vi "Create Test Configuration.vi"(9 "Channel Classification":T1[](array[typedef])=[enum."input data", enum."output data", enum."input data", enum."output data"], 10 "Modbus Type":T2[](array[typedef])=[enum."Holding Registers", enum."Holding Registers", enum."Coils", enum."Coils"], 11 "Data Type":T3[](array[typedef])=[enum."U16", enum."U16", enum."Boolean", enum."Boolean"]) -> (0 "error out":errorcluster, 1 "Names":string[](array[string]), 2 "Channels":refnum<class "Modbus Module Channel.lvclass">[](array[class]), 3 "Module configuration":refnum<class "Modbus Module configuration.lvclass">)   [LabVIEW 2015, in "Modbus Tests.lvlib"]
uses:
  Modbus Tests.lvlib
  module/configuration/Modbus Module configuration.lvclass
  module/module channel/Modbus Module Channel.lvclass
  <vilib>/NI/Tag Bus/tag/Data Type.ctl
  module/module channel/data bank type.ctl
  <vilib>/NI/Tag Bus Module Framework/channel/channel classification.ctl
  <vilib>/NI/Tag Bus/tag/tag descriptor.lvclass/tag descriptor.ctl
  module/module channel/Modbus Module Channel.lvclass/Modbus Module Channel.ctl
  <vilib>/NI/Tag Bus Module Framework/channel/TBM channel.lvclass/TBM channel.ctl
  <vilib>/NI/Tag Bus/tag/write data type.vi
  module/module channel/Write modbus type.vi
  module/module channel/Write starting address.vi
  <vilib>/NI/Tag Bus Module Framework/channel/Write channel classification.vi
  <vilib>/NI/Tag Bus/tag/write tag name.vi
  <vilib>/NI/Configuration Framework/serializable configuration/NISE_CEF_serializable configuration.lvclass
  <vilib>/NI/Tag Bus/tag/tag descriptor.lvclass
  <vilib>/NI/Tag Bus Module Framework/channel/TBM channel.lvclass
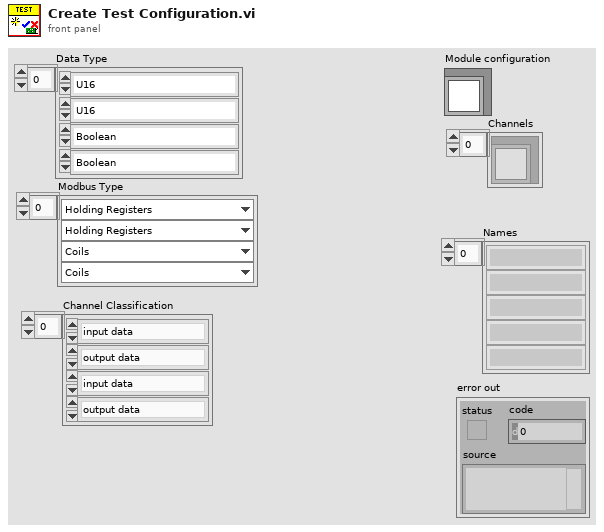
[diagram p1: front panel]
types:
  T1 = typedef "TBM channel.lvclass/channel classification.ctl" = enum16{"input data", "output data", "processing parameter", "processing result"}
  T2 = typedef "Modbus Module Channel.lvclass/data bank type.ctl" = enum16{"Coils", "Discrete Inputs", "Input Registers", "Holding Registers"}
  T3 = typedef "tag bus.lvlib/tag descriptor.lvclass/Data Type.ctl" = enum16{"Double", "Single", "I64", "I32", "I16", "I8", "U64", "U32", "U16", "U8", "Boolean", "String", "Array of Double", "Array of Single", "Array of I64", "Array of I32", "Array of I16", "Array of I8", "Array of U64", "Array of U32", "Array of U16", "Array of U8", "Array of Boolean", "Array of String"}
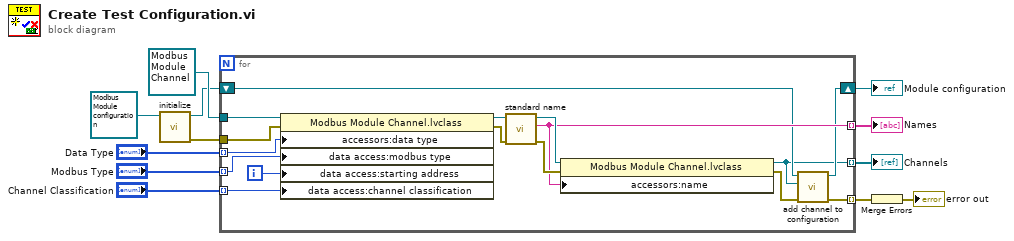
[diagram p0: block diagram]
diagram:
  n1 = call <vilib>:"initialize.vi"("configuration in"=refnum<class "Modbus Module configuration.lvclass"> refnum ("Modbus Module configuration")) -> ("error out"=w3:errorcluster, "configuration out"=w9:refnum<class "Modbus Module configuration.lvclass">)  [unwired: 8 in, 1 out]
  n2 = for {
    tunnel: refnum<class "Modbus Module Channel.lvclass"> refnum ("Modbus Module Channel in") -> [w14]
    tunnel: [w26] -> w10 mode=indexing
    shift-right: [w24] -> w8
    shift-left: w9 -> [w25]
    tunnel: [w23] -> w7 mode=indexing
    tunnel: "Data Type" -> [w22] mode=indexing
    tunnel: [w20] -> w4 mode=indexing
    tunnel: w3 -> [w18]
    tunnel: "Channel Classification" -> [w17] mode=indexing
    tunnel: "Modbus Type" -> [w13] mode=indexing
    i -> [w16]
    n3 = property class="Modbus Module Channel.lvclass"(reference=w14, error in=w18, "accessors:data type"=w22, "data access:modbus type"=w13, "data access:starting address"=w16, "data access:channel classification"=w17) -> (reference out=w15:refnum<class "Modbus Module Channel.lvclass">, error out=w19:errorcluster)
    n4 = call "standard name.vi"("error in"=w19, "Modbus Module Channel in"=w15) -> ("error out"=w27:errorcluster, "standard name"=w26:string, "Modbus Module Channel out"=w28:refnum<class "Modbus Module Channel.lvclass">)  [unwired: 7 in]
    n5 = property class="Modbus Module Channel.lvclass"(reference=w28, error in=w27, "accessors:name"=w26) -> (reference out=w20:refnum<class "Modbus Module Channel.lvclass">, error out=w21:errorcluster)
    n6 = call "add channel to configuration.vi"("error in"=w21, "Modbus Module Channel.lvclass"=w20, "Modbus Slave configuration in"=w25) -> ("error out"=w23:errorcluster, "Modbus Slave configuration out"=w24:refnum<class "Modbus Module configuration.lvclass">)  [unwired: 7 in]
  }
  "Module configuration" <- w8
  "Channels" <- w4
  "Names" <- w10
  n7 = Merge Errors(w7) -> (→"error out":errorcluster)
